vi "initializer_tree_control.vi"(10 "Point":T1, 11 "Parameters Tree":refnum<vi>) -> ()   [LabVIEW 2019]
uses:
  <vilib>/Utility/miscctls.llb/LVPositionTypeDef.ctl
panel:
  # "*******************************************************************\nBiogas Plant Control\n\nAuthor: Paul Zügel\nGCSC-Frankfurt am Main 2020\n\n*******************************************************************"
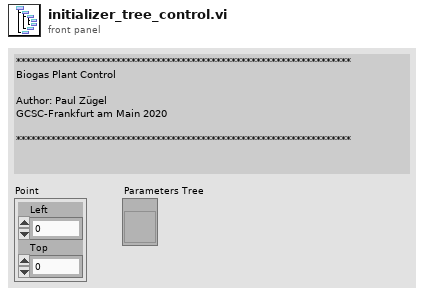
[diagram p1: front panel]
types:
  T1 = typedef "LVPositionTypeDef.ctl" = cluster{"Left":i32, "Top":i32}
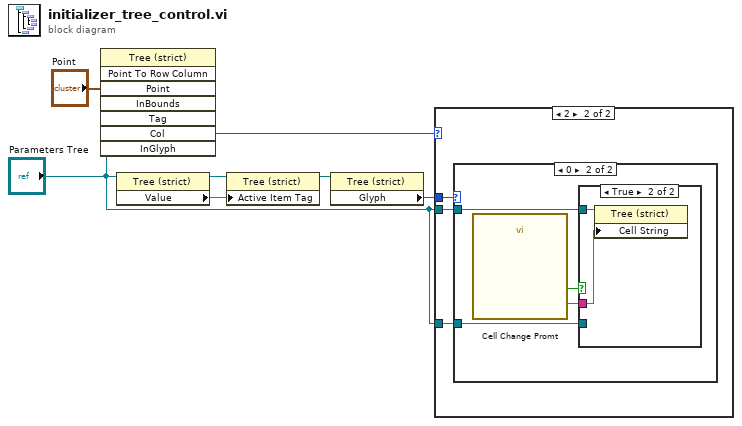
[diagram p0: block diagram]
diagram:
  n1 = invoke on="Invoke Node" class="Tree (strict)" method="Point To Row Column"(reference="Parameters Tree", "Point"="Point") -> ("Col"=w4:i32)  [unwired: 6 in, 7 out]
  n2 = property on="Property Node" class="Tree (strict)"(reference="Parameters Tree") -> (reference out=w7:refnum<vi>, "Value"=w5:string)  [unwired: 1 in, 1 out]
  n3 = property on="Property Node" class="Tree (strict)"(reference=w7, "Active Item Tag"=w5) -> (reference out=w6:refnum<vi>)  [unwired: 1 in, 1 out]
  n4 = property class="Tree (strict)"(reference=w6) -> ("Glyph"=w3:i32)  [unwired: 1 in, 2 out]
  n5 = case shown="2" w4 {
    tunnel: "Parameters Tree" -> [_ w10]
    tunnel: w3 -> [_ w9]
    tunnel: "Parameters Tree" -> [_ w8]
    frame 0, 1, Default {
    }
    frame 2 {
      n6 = case shown="0" w9 {
        tunnel: w10 -> [_ w13]
        tunnel: w8 -> [_ w11]
        frame 15, Default {
        }
        frame 0 {
          n7 = call "Cell Change Promt"() -> ("New Value"=w14:string, "OK"=w12:bool)  [unwired: 17 in, 1 out]
          n8 = case shown="True" w12 {
            tunnel: w14 -> [_ w16]
            tunnel: w13 -> [_ w15]
            tunnel: w11 -> [_ _]
            frame False {
            }
            frame True {
              n9 = property class="Tree (strict)"(reference=w15, "Cell String"=w16) -> ()  [unwired: 1 in, 2 out]
            }
          }
        }
      }
    }
  }
